vi "createInterface.vi"(8 "error in (no error)":errorcluster, 11 "MotorController in":refnum<class "MotorController.lvclass">) -> (0 "error out":errorcluster, 2 "interface object out":refnum<k20>, 3 "MotorController out":refnum<class "MotorController.lvclass">)   [LabVIEW 2018, in "MotorController.lvclass"]
uses:
  MotorController.lvclass
  MotorController.lvclass/MotorController.ctl
  <vilib>/CANopenLib/CANOPEN.llb/CANopen Interface Create.vi
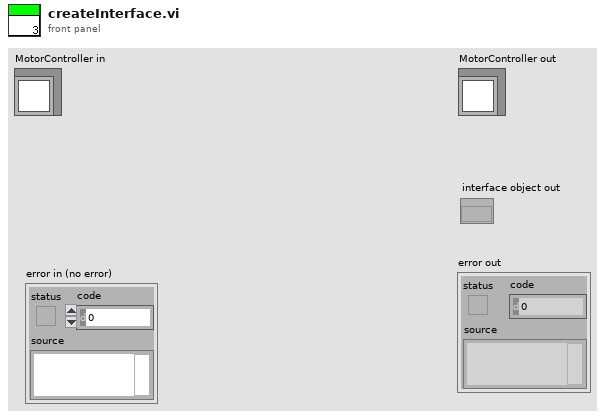
[diagram p1: front panel]
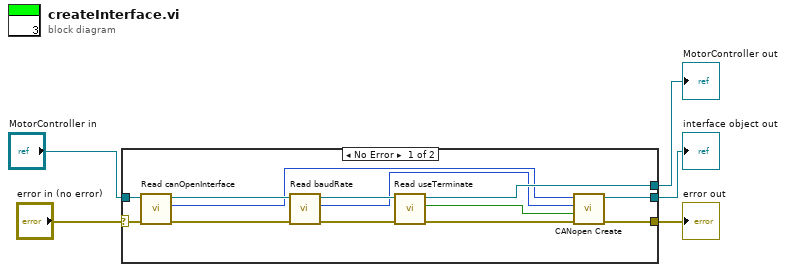
[diagram p0: block diagram]
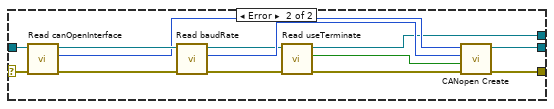
[diagram p2: hidden frame]
diagram:
  n1 = case shown="No Error" "error in (no error)" {
    selector: "error in (no error)" -> [w9 w22]
    tunnel: [w11 w19] -> w4
    tunnel: [w8 w21] -> w2
    tunnel: "MotorController in" -> [w10 w23]
    tunnel: [w12 w20] -> w1
    frame No Error {
      n2 = call "Read canOpenInterface.vi"("error in (no error)"=w9, "MotorController in"=w10) -> ("error out"=w17:errorcluster, "canOpenInterface"=w6:u32, "MotorController out"=w18:refnum<class "MotorController.lvclass">)  [unwired: 7 in]
      n3 = call "Read baudRate.vi"("error in (no error)"=w17, "MotorController in"=w18) -> ("error out"=w15:errorcluster, "baudRate"=w7:u32, "MotorController out"=w16:refnum<class "MotorController.lvclass">)  [unwired: 7 in]
      n4 = call "Read useTerminate.vi"("error in (no error)"=w15, "MotorController in"=w16) -> ("error out"=w13:errorcluster, "useTerminate"=w14:bool, "MotorController out"=w8:refnum<class "MotorController.lvclass">)  [unwired: 7 in]
      n5 = call-poly <vilib>:"CANopen Create.vi"("error in (no error)"=w13, "termination? (F)"=w14, "baud rate"=w7, "interface name"=w6) -> ("error out"=w11:errorcluster, "interface object out"=w12:refnum<k20>)  [unwired: 6 in]
    }
    frame Error {
      n6 = call "Read canOpenInterface.vi"("error in (no error)"=w22, "MotorController in"=w23) -> ("error out"=w30:errorcluster, "canOpenInterface"=w29:u32, "MotorController out"=w31:refnum<class "MotorController.lvclass">)  [unwired: 7 in]
      n7 = call "Read baudRate.vi"("error in (no error)"=w30, "MotorController in"=w31) -> ("error out"=w26:errorcluster, "baudRate"=w28:u32, "MotorController out"=w27:refnum<class "MotorController.lvclass">)  [unwired: 7 in]
      n8 = call "Read useTerminate.vi"("error in (no error)"=w26, "MotorController in"=w27) -> ("error out"=w24:errorcluster, "useTerminate"=w25:bool, "MotorController out"=w21:refnum<class "MotorController.lvclass">)  [unwired: 7 in]
      n9 = call-poly <vilib>:"CANopen Create.vi"("error in (no error)"=w24, "termination? (F)"=w25, "baud rate"=w28, "interface name"=w29) -> ("error out"=w19:errorcluster, "interface object out"=w20:refnum<k20>)  [unwired: 6 in]
    }
  }
  "error out" <- w4
  "MotorController out" <- w2
  "interface object out" <- w1
